vi "Fill DataTable (double array).vi"(6 "modeling type (Continuous)":enum16{"Continuous", "Ordinal", "Nominal"}(ring), 8 "error in (no error)":errorcluster, 9 "columns name":string[](array[string]), 10 "columns data":dbl[][](array[numeric]), 11 "JMP DataTable":refnum<k7>) -> (0 "error out":errorcluster, 3 "JMP DataTable out":refnum<k7>)   [LabVIEW 2019, in "JMP Automation.lvlib"]
doc: "Add columns with their coresponding data to a DataDable"
uses:
  <instrlib>/LV_JMP_bridge/JMP Automation.lvlib
  <instrlib>/LV_JMP_bridge/JMP Column.ctl
  <instrlib>/LV_JMP_bridge/JMP Column Header.ctl
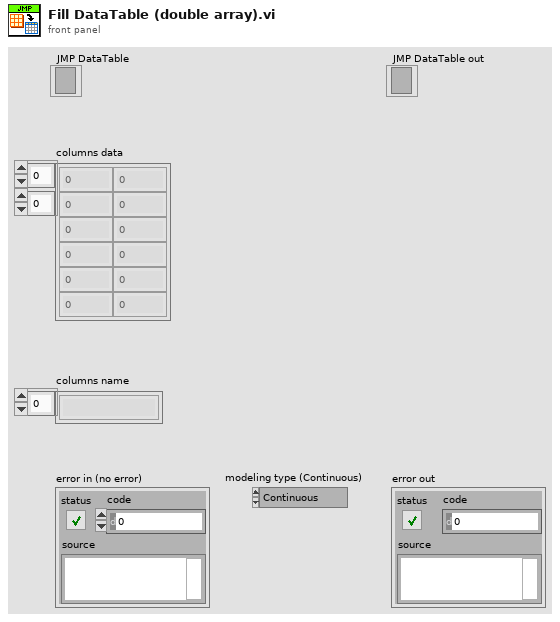
[diagram p1: front panel]
types:
  T1 = typedef "JMP Automation.lvlib/JMP Column.ctl" = cluster{"Header":T2, "Data":variant[]}
  T2 = typedef "JMP Automation.lvlib/JMP Column Header.ctl" = cluster{"Column Name":string, "Lock":bool, "Data Type":enum16{"Unknown", "Numeric", "Character", "RowState"}, "Modeling Type":enum16{"Continuous", "Ordinal", "Nominal"}}
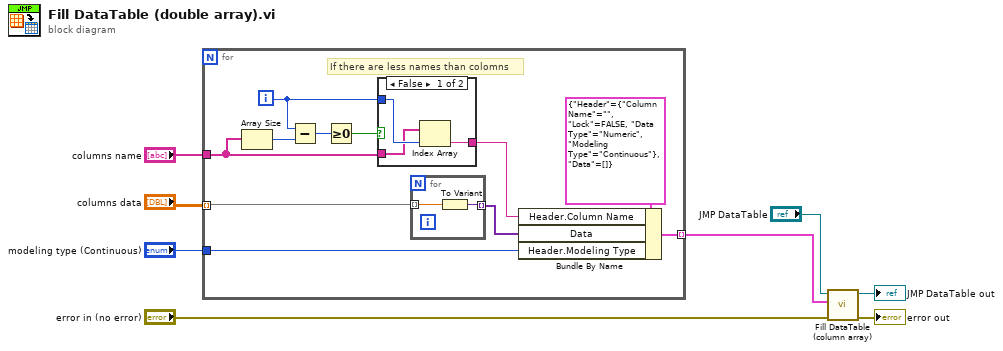
[diagram p0: block diagram]
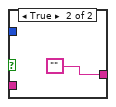
[diagram p2: hidden frame]
diagram:
  n1 = for {
    tunnel: "columns data" -> [w10] mode=indexing
    tunnel: "modeling type (Continuous)" -> [w18]
    tunnel: [w17] -> w3 mode=indexing
    tunnel: "columns name" -> [w14]
    i -> [w11]
    # "If there are less names than colomns"
    n2 = Array Size(array=w14) -> (size(s)=w12:i32)
    n3 = Subtract(x=w11, y=w12) -> (x-y=w16:i32)
    n4 = Greater Or Equal To 0?(x=w16) -> (x >= 0?=w15:bool)
    n5 = case shown="False" w15 {
      tunnel: w11 -> [w24 _]
      tunnel: w14 -> [w23 _]
      tunnel: [w22 ""] -> w13
      frame False {
        n6 = Index Array(array=w23, index=w24) -> (element=w22:string)
      }
      frame True {
      }
    }
    n7 = for {
      tunnel: w10 -> [w21] mode=indexing
      tunnel: [w20] -> w9 mode=indexing
      n8 = To Variant(anything=w21) -> (Variant=w20:variant)
    }
    n9 = Bundle By Name(cluster=T1 {"Header"={"Column Name"="", "Lock"=FALSE, "Data Type"=enum."Numeric", "Modeling Type"=enum."Continuous"}, "Data"=[]} ("JMP Column"), "Header.Column Name"=w13, "Data"=w9, "Header.Modeling Type"=w18) -> (w17:T1)
  }
  n10 = call <instrlib>:"Fill DataTable (column array).vi"("error in (no error)"="error in (no error)", "columns"=w3, "JMP DataTable"="JMP DataTable") -> ("error out"=→"error out":errorcluster, "JMP data table out"=→"JMP DataTable out":refnum<k7>)  [unwired: 7 in]
